vi "How I Am.vi"() -> ()   [LabVIEW 2010]
doc: "This SubVI takes clean How sense data from the Midbrain and layers perception onto it to be passed to the THINK processes in the Forebrain"
uses:
  5.0-Global.vi
  6-OCU Neurons/CommonIndicators.ctl
  <vilib>/ptbypt/NI_PtbyPt.lvlib
  4-High Neurons/How Sensor Typedef.ctl
panel:
  out "5.3.3 How Am I? Sensor":T1
  out "How?":bool
  # "This SubVI adds \nperception onto the\nHow data comming\nfrom the Midbrain"
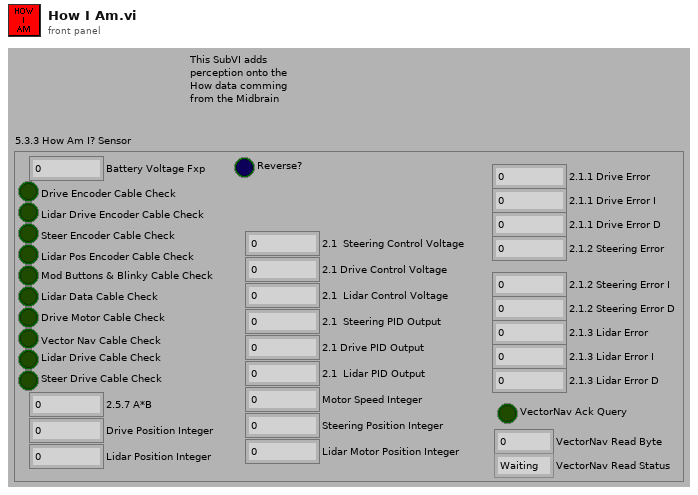
[diagram p1: front panel]
types:
  T1 = typedef "How Sensor Typedef.ctl" = cluster{"Motor Speed Integer":i32, "Drive Position Integer":i32, "Lidar Position Integer":i32, "Lidar Motor Position Integer":i32, "Steering Position Integer":i32, "Battery Voltage Fxp":dbl, "Drive Encoder Cable Check":bool, "Lidar Drive Encoder Cable Check":bool, "Steer Encoder Cable Check":bool, "Lidar Pos Encoder Cable Check":bool, "Mod Buttons & Blinky Cable Check":bool, "Lidar Data Cable Check":bool, "Drive Motor Cable Check":bool, "Vector Nav Cable Check":bool, "Lidar Drive Cable Check":bool, "Steer Drive Cable Check":bool, "Reverse?":bool, "2.1  Steering Control Voltage":dbl, "2.1 Drive Control Voltage":dbl, "2.1  Lidar Control Voltage":dbl, "2.5.7 A*B":dbl, "2.1  Steering PID Output":dbl, "2.1 Drive PID Output":dbl, "2.1  Lidar PID Output":dbl, "2.1.1 Drive Error":dbl, "2.1.1 Drive Error I":dbl, "2.1.1 Drive Error D":dbl, "2.1.2 Steering Error":dbl, "2.1.2 Steering Error I":dbl, "2.1.2 Steering Error D":dbl, "2.1.3 Lidar Error":dbl, "2.1.3 Lidar Error I":dbl, "2.1.3 Lidar Error D":dbl, "VectorNav Ack Query":bool, "VectorNav Read Byte":u8, "VectorNav Read Status":enum16{"Waiting", "Reading", "Done"}}
  T2 = typedef "CommonIndicators.ctl" = cluster{"Speed":dbl, " Heading":cluster{dbl, dbl}, "MissionTime":dbl, "Battery":dbl, "MAP":bool, "LIDAR":bool, "ManualMissionMap":picture, "ManualModeLIDAR":picture, "ManualModeStop":bool, "How?":bool, "Where?":bool, "What?":bool, "ActManual":bool, "CollisionLight ":bool, "Ready":bool}
  T3 = cluster{"X (Current)":dbl, "Y (Current) ":dbl, "Heading":dbl, "Steering Angle":dbl}
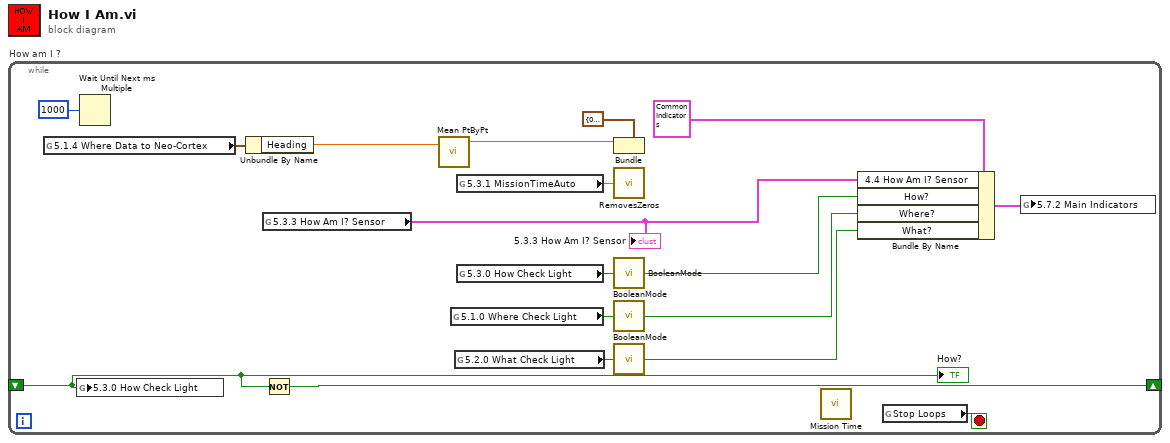
[diagram p0: block diagram]
diagram:
  n1 = while "How am I ?" {
    shift-right: [w17] -> _
    shift-left: _ -> [w15]
    stop <- w16 stop-if-true
    n2 = global read "5.0-Global.vi" "5.1.4 Where Data to Neo-Cortex"() -> (w7:T3)
    n3 = global write "5.0-Global.vi" "5.3.0 How Check Light"(w15) -> ()
    n4 = Wait Until Next ms Multiple(millisecond multiple=u32 1000 ("milliseconds to wait")) -> ()  [unwired: 1 out]
    n5 = Unbundle By Name(w7) -> ("Heading"=w9:dbl)
    n6 = global read "5.0-Global.vi" "5.3.3 How Am I? Sensor"() -> (w1:T1)
    "5.3.3 How Am I? Sensor" <- w1
    n7 = Not(x=w15) -> (.not. x?=w17:bool)
    n8 = call <vilib>:"Mean PtByPt.vi"("x"=w9) -> ("mean"=w14:dbl)  [unwired: 3 in, 1 out]
    n9 = global read "5.0-Global.vi" "5.1.0 Where Check Light"() -> (w11:bool)
    n10 = global read "5.0-Global.vi" "5.2.0 What Check Light"() -> (w12:bool)
    n11 = global read "5.0-Global.vi" "5.3.1 MissionTimeAuto"() -> (w13:dbl)
    n12 = global read "5.0-Global.vi" "5.3.0 How Check Light"() -> (w10:bool)
    n13 = Bundle(cluster=cluster{dbl, dbl} {0.0, 0.0} ("Heading"), w14) -> ()  [unwired: 1 in, 1 out]
    n14 = call "RemovesZeros.vi"("5.3.1 MissionTimeAuto 2"=w13) -> ()  [unwired: 1 out]
    n15 = call "BooleanMode.vi"("5.3.0 How Check Light  2"=w10) -> ("5.3.0 How Check Light"=w4:bool)
    n16 = call "BooleanMode.vi"("5.3.0 How Check Light  2"=w11) -> ("5.3.0 How Check Light"=w3:bool)
    n17 = call "BooleanMode.vi"("5.3.0 How Check Light  2"=w12) -> ("5.3.0 How Check Light"=w2:bool)
    n18 = call "Mission Time.vi"() -> ()  [unwired: 1 out]
    n19 = Bundle By Name(cluster=T2 {"Speed"=0.0, " Heading"={0.0, 0.0}, "MissionTime"=0.0, "Battery"=0.0, "MAP"=FALSE, "LIDAR"=FALSE, "ManualMissionMap"=bytes[0], "ManualModeLIDAR"=bytes[0], "ManualModeStop"=FALSE, "How?"=FALSE, "Where?"=FALSE, "What?"=FALSE, "ActManual"=FALSE, "CollisionLight "=FALSE, "Ready"=FALSE} ("5.7.2 Main Indicators"), "4.4 How Am I? Sensor"=w1, "How?"=w4, "Where?"=w3, "What?"=w2) -> (w5:T2)
    n20 = global read "5.0-Global.vi" "Stop Loops"() -> (w16:bool)
    n21 = global write "5.0-Global.vi" "5.7.2 Main Indicators"(w5) -> ()
    "How?" <- w15
  }
